vi "Frameless Modal FP Remove Border.vi"(11 "VI引用":refnum<vi>) -> ()   [LabVIEW 2020]
uses:
  user32.dll
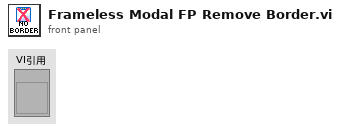
[diagram p1: front panel]
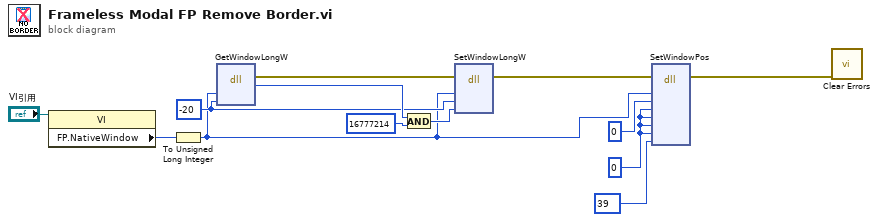
[diagram p0: block diagram]
diagram:
  w4 = 0 ("x")
  w9 = -20
  n1 = property class="VI"(reference="VI引用") -> ("FP.NativeWindow"=w13:u64)  [unwired: 1 in, 2 out]
  n2 = To Unsigned Long Integer(number=w13) -> (unsigned 32bit integer=w6:u32)
  n3 = dll-call lib="user32.dll" fn="GetWindowLongW"("hwnd"=w6, "index"=w9) -> (error out=w10:errorcluster, "返回类型"=w12:i32)  [unwired: 5 in, 1 out]
  n4 = And(x=w12, y=16777214) -> (x .and. y?=w8:i32)
  n5 = dll-call lib="user32.dll" fn="SetWindowLongW"(error in=w10, "hwnd"=w6, "index"=w9, "newStyle"=w8) -> (error out=w7:errorcluster)  [unwired: 6 in, 1 out]
  n6 = dll-call lib="user32.dll" fn="SetWindowPos"(error in=w7, "hwnd"=w6, "InsertAfter"=u32 0, "x"=w4, "y"=w4, "cx"=w4, "cy"=w4, "flag"=u32 39) -> (error out=w1:errorcluster)  [unwired: 10 in, 1 out]
  n7 = call <vilib>:"Clear Errors.vi"("error in (no error)"=w1) -> ()  [unwired: 5 in, 2 out]
